vi "Labview4_subVI.vi"(4 "Cneg":dbl, 6 "Vneg":dbl, 7 "Vpos":dbl, 9 "Boolean":bool, 10 "Cpos":dbl, 11 "output y(t)":dbl) -> (3 "Numeric":dbl)   [LabVIEW 2016]
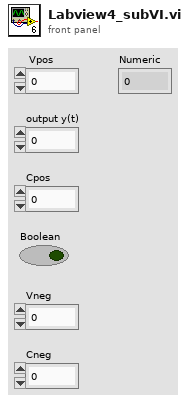
[diagram p1: front panel]
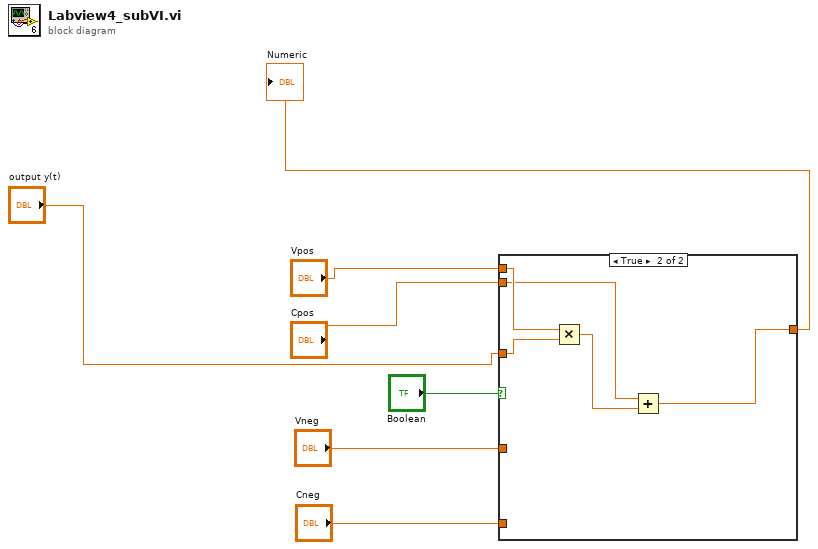
[diagram p0: block diagram]
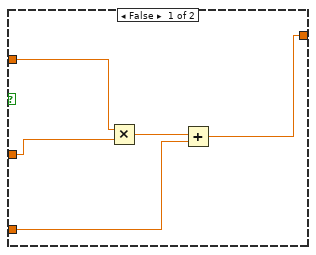
[diagram p2: hidden frame]
diagram:
  n1 = case shown="True" "Boolean" {
    tunnel: "Vpos" -> [_ w17]
    tunnel: "Cpos" -> [_ w14]
    tunnel: "Vneg" -> [w11 _]
    tunnel: "Cneg" -> [w9 _]
    tunnel: "output y(t)" -> [w12 w16]
    tunnel: [w8 w13] -> w7
    frame False {
      n2 = Multiply ("Multiply 2")(x=w12, y=w11) -> (x*y=w10:dbl)
      n3 = Add ("Add 2")(x=w10, y=w9) -> (x+y=w8:dbl)
    }
    frame True {
      n4 = Multiply(x=w17, y=w16) -> (x*y=w15:dbl)
      n5 = Add(x=w14, y=w15) -> (x+y=w13:dbl)
    }
  }
  "Numeric" <- w7
